vi "EXCOM-28.vi"(0 "VISA resource name":refnum<visa-resource-name>, 5 "Error IN":errorcluster, 6 "Bool Refnum":refnum<vi>) -> (14 "VISA resource name dup":refnum<visa-resource-name>, 15 "NORA":dbl format="%<%H:%M:%S%0u>t", 16 "NODEC":dbl format="%<%H:%M:%S%0u>t", 17 "DEC":dbl format="%.2f", 18 "HA":dbl format="%.2f", 19 "Error OUT":errorcluster)   [LabVIEW 2011]
panel:
  out "TCS C actif":bool
  out "RA":dbl format="%<%H:%M:%S%0u>t"
  out "OK Done":bool
  out "Q String":string
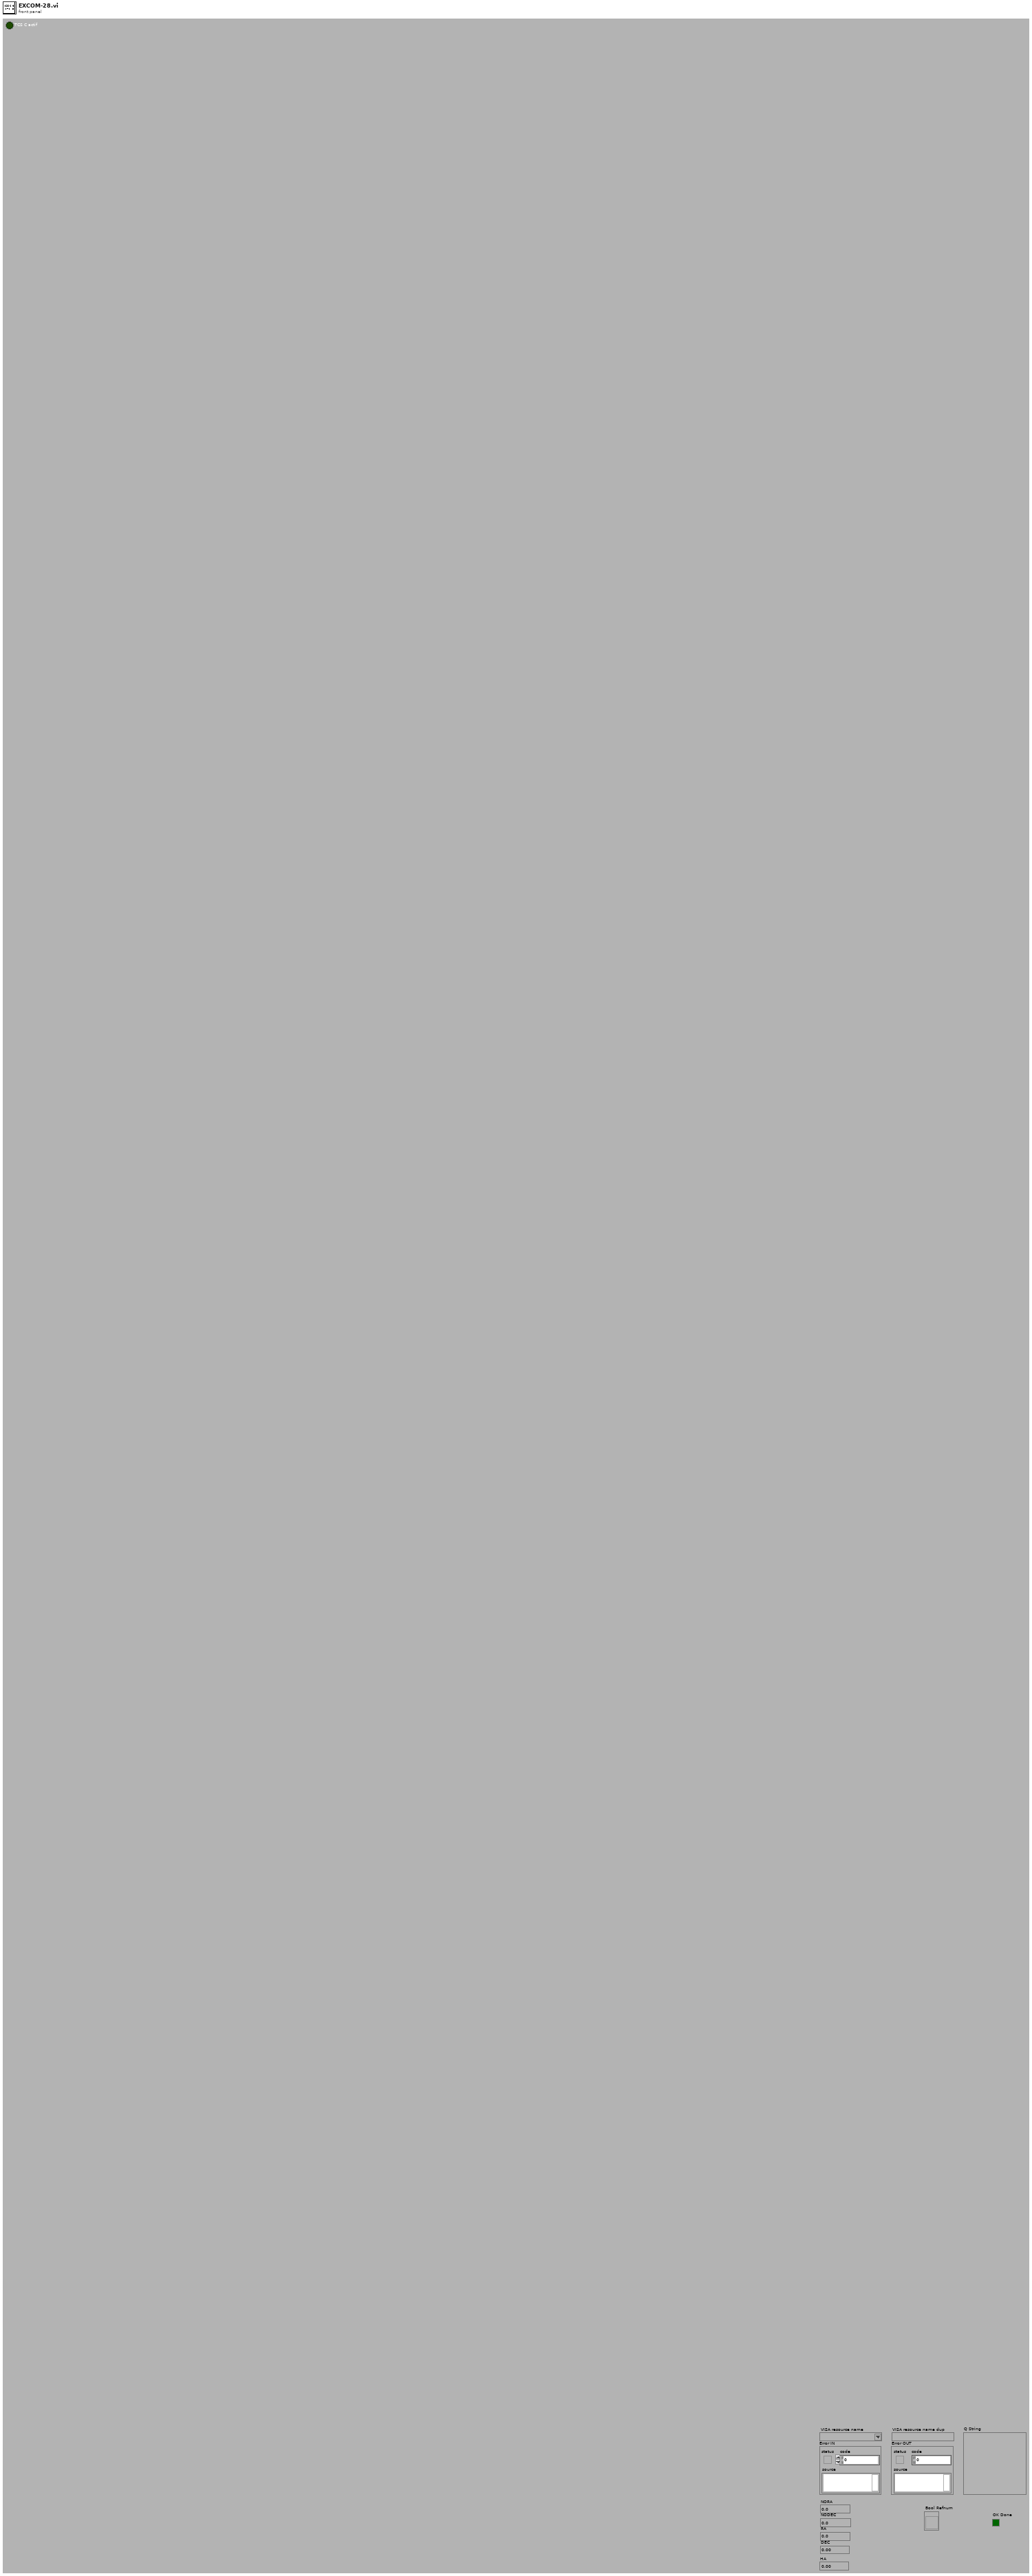
[diagram p1: front panel]
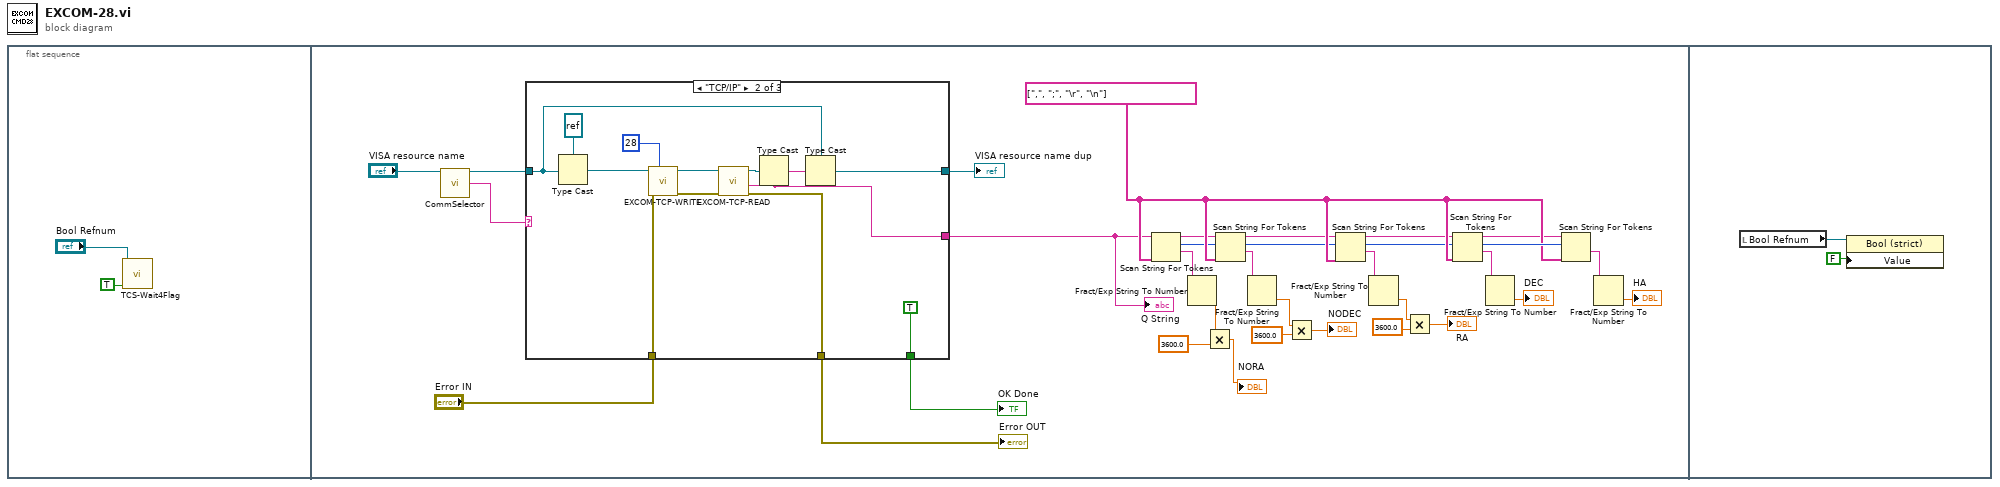
[diagram p0: block diagram]
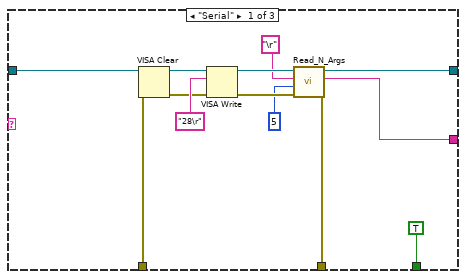
[diagram p2: hidden frame]
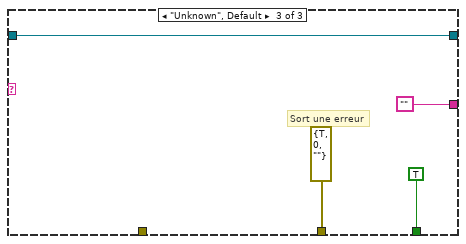
[diagram p3: hidden frame]
diagram:
  n1 = flat-sequence {
    frame #0 {
      n2 = call "TCS-Wait4Flag.vi"("Raise Flag ?"=TRUE, "Ctl Refnum IN"="Bool Refnum") -> ()  [unwired: 8 in, 2 out]
    }
    frame #1 {
      w27 = string[] [",", ";", "\r", "\n"] ("delimiters (\\s,\\t,\\r,\\n)")
      n3 = call "CommSelector.vi"("VISA resource name"="VISA resource name") -> ("VISA resource name"=w30:refnum<visa-resource-name>, "CommType"=w29:string)  [unwired: 13 in]
      n4 = case shown="\"TCP/IP\"" w29 {
        tunnel: w30 -> [w40 w51 w63]
        tunnel: [TRUE ("OK Done") TRUE ("OK Done") TRUE ("OK Done")] -> w35
        tunnel: [w47 w55 errorcluster {"status"=TRUE, "code"=0, "source"=""} ("error out")] -> w34
        tunnel: [w41 w50 w63] -> w33
        tunnel: "Error IN" -> [w38 w59 _]
        tunnel: [w36 w53 ""] -> w3
        frame "Serial" {
          n5 = VISA Clear(VISA resource name=w40, error in (no error)=w38) -> (VISA resource name out=w39:refnum<visa-resource-name>, error out=w37:errorcluster)
          n6 = VISA Write(VISA resource name=w39, write buffer="28\r" ("String to Send"), error in (no error)=w37) -> (VISA resource name out=w45:refnum<visa-resource-name>, error out=w46:errorcluster)  [unwired: 1 out]
          n7 = call "Read_N_Args.vi"("Error IN"=w46, "Nb_Args"=5, "Arg_Char"="\r", "VRN IN"=w45) -> ("Error OUT"=w47:errorcluster, "Answer"=w36:string, "VRN OUT"=w41:refnum<visa-resource-name>)  [unwired: 4 in, 1 out]
        }
        frame "TCP/IP" {
          n8 = Type Cast(type=refnum<k5> refnum ("connection ID out"), x=w51) -> (*(type *) &x=w60:refnum<k5>)
          n9 = call "EXCOM-TCP-WRITE.vi"("Commande #"=28, "Error IN"=w59, "connection ID"=w60) -> ("Error OUT"=w56:errorcluster, "connection ID out"=w57:refnum<k5>)  [unwired: 4 in, 2 out]
          n10 = call "EXCOM-TCP-READ.vi"("Error In"=w56, "connection ID"=w57) -> ("Error Out"=w55:errorcluster, "Response"=w53:string, "CID Out"=w54:refnum<k5>)  [unwired: 5 in]
          n11 = Type Cast(type=w53, x=w54) -> (*(type *) &x=w52:string)
          n12 = Type Cast(type=w51, x=w52) -> (*(type *) &x=w50:refnum<visa-resource-name>)
        }
        frame "Unknown", Default {
          # "Sort une erreur"
        }
      }
      "VISA resource name dup" <- w33
      "OK Done" <- w35
      "Error OUT" <- w34
      "Q String" <- w3
      n13 = Scan String For Tokens(6:w27, 9:w3) -> (1:w10:string, 2:w9:i32, 3:w8:string)  [unwired: 4 in, 1 out]
      n14 = Fract/Exp String To Number(string=w10) -> (number=w11:dbl)  [unwired: 3 in, 1 out]
      n15 = Multiply(x=w11, y=3600.0) -> (x*y=→"NORA":dbl)
      n16 = Scan String For Tokens(6:w27, 8:w9, 9:w8) -> (1:w22:string, 2:w6:i32, 3:w7:string)  [unwired: 3 in, 1 out]
      n17 = Fract/Exp String To Number(string=w22) -> (number=w18:dbl)  [unwired: 3 in, 1 out]
      n18 = Multiply(x=w18, y=3600.0) -> (x*y=→"NODEC":dbl)
      n19 = Scan String For Tokens(6:w27, 8:w6, 9:w7) -> (1:w16:string, 2:w4:i32, 3:w5:string)  [unwired: 3 in, 1 out]
      n20 = Fract/Exp String To Number(string=w16) -> (number=w20:dbl)  [unwired: 3 in, 1 out]
      n21 = Multiply(x=w20, y=3600.0) -> (x*y=→"RA":dbl)
      n22 = Scan String For Tokens(6:w27, 8:w4, 9:w5) -> (1:w17:string, 2:w28:i32, 3:w26:string)  [unwired: 3 in, 1 out]
      n23 = Fract/Exp String To Number(string=w17) -> (number=→"DEC":dbl)  [unwired: 3 in, 1 out]
      n24 = Scan String For Tokens(6:w27, 8:w28, 9:w26) -> (1:w25:string)  [unwired: 3 in, 3 out]
      n25 = Fract/Exp String To Number(string=w25) -> (number=→"HA":dbl)  [unwired: 3 in, 1 out]
    }
    frame #2 {
      n26 = local read "Bool Refnum"() -> (w66:refnum<vi>)
      n27 = property class="Bool (strict)"(reference=w66, "Value"=FALSE) -> ()  [unwired: 1 in, 2 out]
    }
  }
